vi "Customize VI Window.vi"() -> ()   [LabVIEW 2009]
doc: "Ce VI illustre les méthodes et les propriétés de VI Serveur : afficher barre de menus, barre de titre visible, transparence du VI et centrage du VI."
panel:
  in  "Centrer":bool
  in  "stop":bool
  in  "VI transparent ?":bool
  in  "Barre de titre visible ?":bool
  in  "Barre de menus visible ?":bool
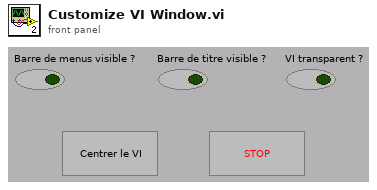
[diagram p1: front panel]
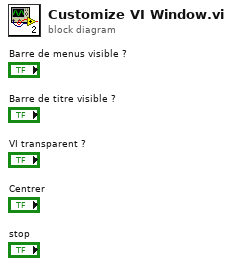
[diagram p0: block diagram]
diagram:
